vi "正向过零（I32）.vi"(2 "输入":i32, 3 "复位":bool) -> (7 "正向过零":bool)   [LabVIEW 2012]
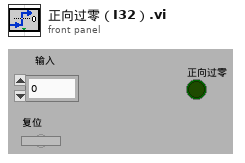
[diagram p1: front panel]
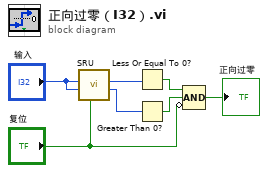
[diagram p0: block diagram]
diagram:
  n1 = call-poly "SRU.vi"("复位"="复位", "初始值"="输入", "输入"="输入") -> ("本次值"=w5:i32, "上次值"=w6:i32)  [unwired: 6 in, 1 out]
  n2 = Less Or Equal To 0?(x=w6) -> (x <= 0?=w4:bool)
  n3 = Greater Than 0?(x=w5) -> (x > 0?=w3:bool)
  n4 = Compound Arithmetic op=AND(w4, w3, invert "复位") -> (→"正向过零":bool)
